vi "myRIO_BRig_RT_dataBlock_nTrials__R.vi"() -> (2 "output_nTrials__R":i32)   [LabVIEW 2014]
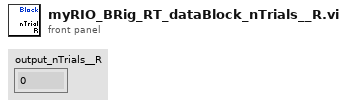
[diagram p1: front panel]
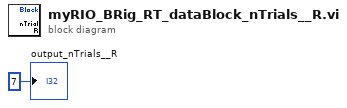
[diagram p0: block diagram]
diagram:
  "output_nTrials__R" <- 7 ("output_iBlock")
